vi "21_Add and Subtract using Case Structure.vi"() -> ()   [LabVIEW 2018]
panel:
  in  "Push Button":bool
  out "Result":dbl
  in  "B":dbl
  in  "A":dbl
  # "Develop a HMI to perform addition and subtraction using case structure\nif switch is on: Addition\nif switch is off: Subtraction"
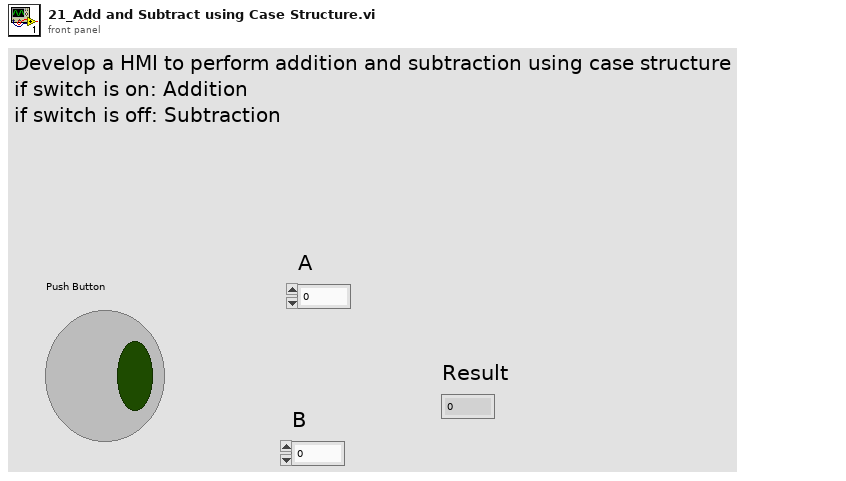
[diagram p1: front panel]
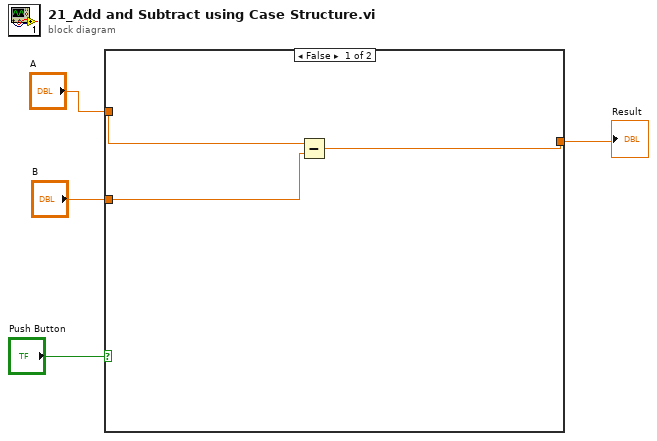
[diagram p0: block diagram]
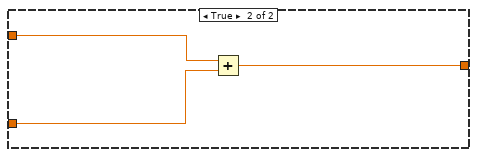
[diagram p2: hidden frame]
diagram:
  n1 = case shown="False" "Push Button" {
    tunnel: "A" -> [w7 w10]
    tunnel: "B" -> [w6 w9]
    tunnel: [w5 w8] -> w1
    frame False {
      n2 = Subtract(x=w7, y=w6) -> (x-y=w5:dbl)
    }
    frame True {
      n3 = Add(x=w10, y=w9) -> (x+y=w8:dbl)
    }
  }
  "Result" <- w1
